vi "Analiza Spectralamodificat.vi"() -> ()   [LabVIEW 2020]
uses:
  <vilib>/express/express analysis/Spectral/Block/exnSpectralBlock spectral measurements RMS poly.vi
  <vilib>/express/express analysis/Spectral/Block/exnSpectralBlock spectral measurements RMS WFM.vi
  <vilib>/express/express analysis/Spectral/XNode/ExpressSpectralMeasurementsBlockNode.xnode
  <vilib>/measure/NI_MAPro.lvlib
  <vilib>/measure/NI_MABase.lvlib
panel:
  out "Waveform Graph 1":waveform(dbl)(graph)
  in  "Durata Semnal":dbl
  in  "Esantioane":dbl
  in  "Tip Semnal Baza/Formula":bool
  in  "Index Formula":dbl
  in  "Formula":string[](array[string])
  in  "square wave duty cycle (%)":dbl=50.0 format="%0.2f"
  out "Waveform Graph 2":cluster{"f0":dbl, "df":dbl, "magnitude":dbl[]}(graph)
  in  "Amplitudine":i64(slide) scale=0.0..10.0
  in  "Frecventa":i64(slide) min=1 max=1000 step=1 scale=1.0..1000.0
  in  "stop":bool
  in  "Tipul Semnalului":T1(ring)
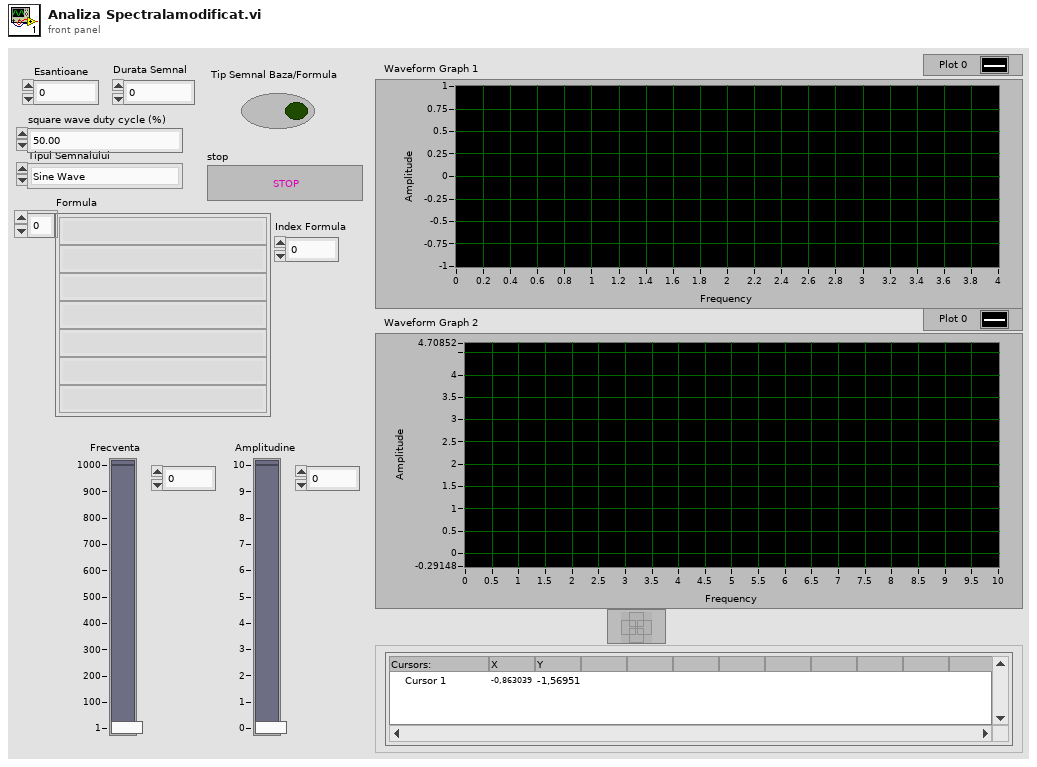
[diagram p1: front panel]
types:
  T1 = enum16{"Sine Wave", "Triangle Wave", "Square Wave", "Sawtooth Wave"}
  T2 = cluster{"averaging mode":u16, "weighting mode":u16, "number of averages":u32}
  T3 = cluster{"dB On (F)":bool, "unwrap phase (F)":bool, "convert to degree (F)":bool}
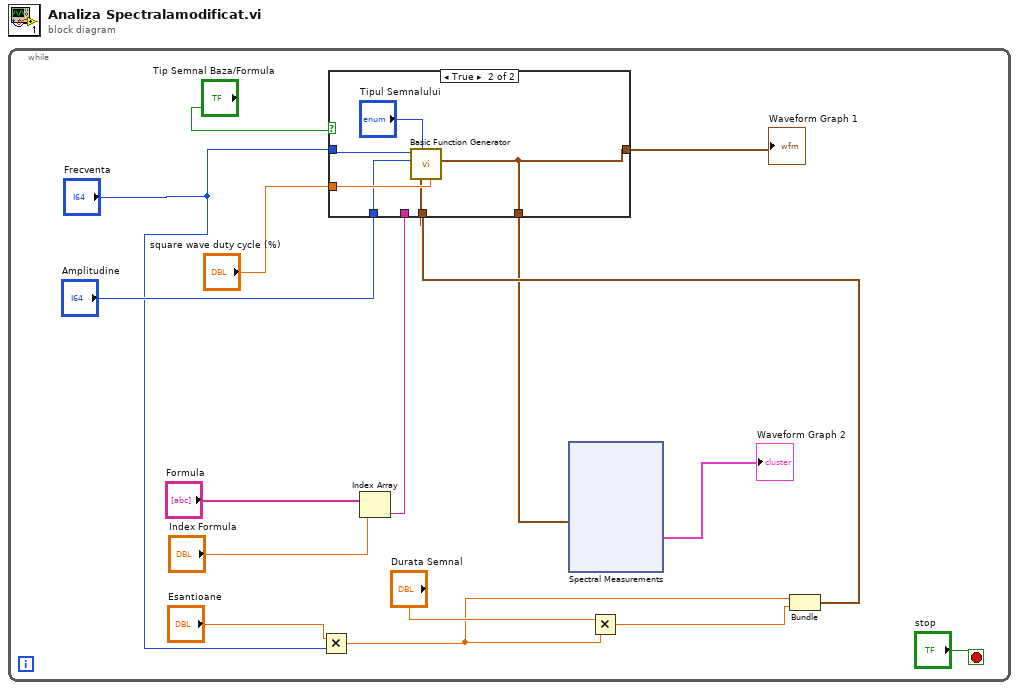
[diagram p0: block diagram]
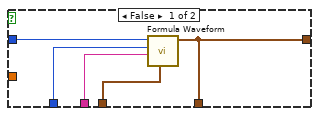
[diagram p2: hidden frame]
diagram:
  n1 = while {
    stop <- "stop" stop-if-true
    n2 = Multiply(x="Esantioane", y="Frecventa") -> (x*y=w6:dbl)
    n3 = Index Array(array="Formula", index="Index Formula") -> (element=w10:string)
    n4 = Multiply(x="Durata Semnal", y=w6) -> (x*y=w5:dbl)
    n5 = Bundle(w6, w5) -> (w3:cluster{dbl, dbl})  [unwired: 1 in]
    n6 = case shown="True" "Tip Semnal Baza/Formula" {
      tunnel: "square wave duty cycle (%)" -> [_ w27]
      tunnel: "Amplitudine" -> [w21 w26]
      tunnel: w10 -> [w20 _]
      tunnel: [w19 w22] -> w4
      tunnel: [w19 w22] -> w1
      tunnel: w3 -> [w18 w23]
      tunnel: "Frecventa" -> [w17 w25]
      frame False {
        n7 = call <vilib>:"Formula Waveform.vi"("sampling info"=w18, "formula"=w20, "amplitude"=w21, "frequency"=w17) -> ("signal out"=w19:waveform(dbl))  [unwired: 6 in, 1 out]
      }
      frame True {
        n8 = call <vilib>:"Basic Function Generator.vi"("square wave duty cycle (%)"=w27, "sampling info"=w23, "signal type"="Tipul Semnalului", "amplitude"=w26, "frequency"=w25) -> ("signal out"=w22:waveform(dbl))  [unwired: 4 in, 2 out]
      }
    }
    "Waveform Graph 1" <- w4
    n9 = xnode "Spectral Measurements"("Signals"=w1) -> ("FFT - (RMS)"=→"Waveform Graph 2":cluster{"f0":dbl, "df":dbl, "magnitude":dbl[]})  [unwired: 1 in, 2 out]
  }
